vi "Calculate Counter And Protections Main Incoming.vi"(0 "Incoming Frames":T5[](array[typedef]) {"Protection Configurations"."CRC Channels"."Data Type" items=["Signed", "Unsigned", "IEEE Float"]}, 1 "TimeStamp.Ref":T1, 2 "TimeDiff.Ref":T1, 5 "Incoming Values in":T4, 7 "data":T2[](array[typedef]) {"payload" format="%x"; "timestamp" format="%<%.7X\n%x>T"; "type" items=["CAN Data"=0, "CAN Remote"=1, "CAN Bus Error"=2, "CAN 2.0 Data"=8, "CAN FD Data"=16, "CAN FD+BRS Data"=24, "J1939 Data"=192, "Delay"=224, "Log Trigger"=225, "Start Trigger"=226]; "identifier" format="%x"}, 11 "error in (no error)":errorcluster, 12 "IncomingSignals.Ref":T1, 13 "CtrandProtctnVld.Ref":T1, 14 "IncomingProtCtr.Ref":T1) -> (6 "Incoming Values out":T4, 15 "error out":errorcluster)   [LabVIEW 2024, in "Protection and Counter Support Engine.lvlib"]
uses:
  Protection and Counter Support Engine.lvlib
  Types/RT Frame Incoming Values.ctl
  Types/RT Frame Settings.ctl
  Shared/Types/Exported Frame Type.ctl
  Types/RT Protection Configuration.ctl
  Shared/Types/Protection Type.ctl
  Shared/Types/XNET Signal Configuration.ctl
  Shared/Types/Exported Counter Settings.ctl
  Shared/Types/Exported Event Trigger Type.ctl
  <vilib>/xnet/xnet.llb/XNET Frame CAN.ctl
  <vilib>/xnet/xnet.llb/XNET Frame Type CAN.ctl
  <vilib>/NI/NIVS Inline Async API/_Data Access Engine/Data Access Engine/Types/Write.DVR.ctl
  <vilib>/NI/NIVS Inline Async API/_Data Access Engine/Access Type Classes/Write/Write.lvclass
  <vilib>/NI/NIVS Inline Async API/_Data Access Engine/Access Type Classes/Write/Write.lvclass/Write.ctl
  <vilib>/NI/NIVS Inline Async API/_Data Access Engine/Data Access Engine/Methods/Write.Data.vi
  Calculate Protection Value.vi
  <vilib>/NI/NIVS Inline Async API/_Data Access Engine/Access Type Classes/Write/Write.ProcessData.vi
  Get Protection Signals.vi
  <vilib>/NI/NIVS Inline Async API/_Data Access Engine/Access Type Classes/Write/Write.Buffer.vi
  <vilib>/NI/NIVS Inline Async API/_Data Access Engine/Access Type Classes/Write/Write.Commit.vi
  <vilib>/xnet/xnet.llb/XNET Convert (Frame CAN to Signal).vi
  <vilib>/xnet/xnet.llb/XNET Convert (Signal to Frame Raw).vi
  <vilib>/NI/NIVS Inline Async API/_Data Access Engine/Data Access Engine/Data Access Engine.lvclass
  Shared/Protection and Counter Support Shared.lvlib
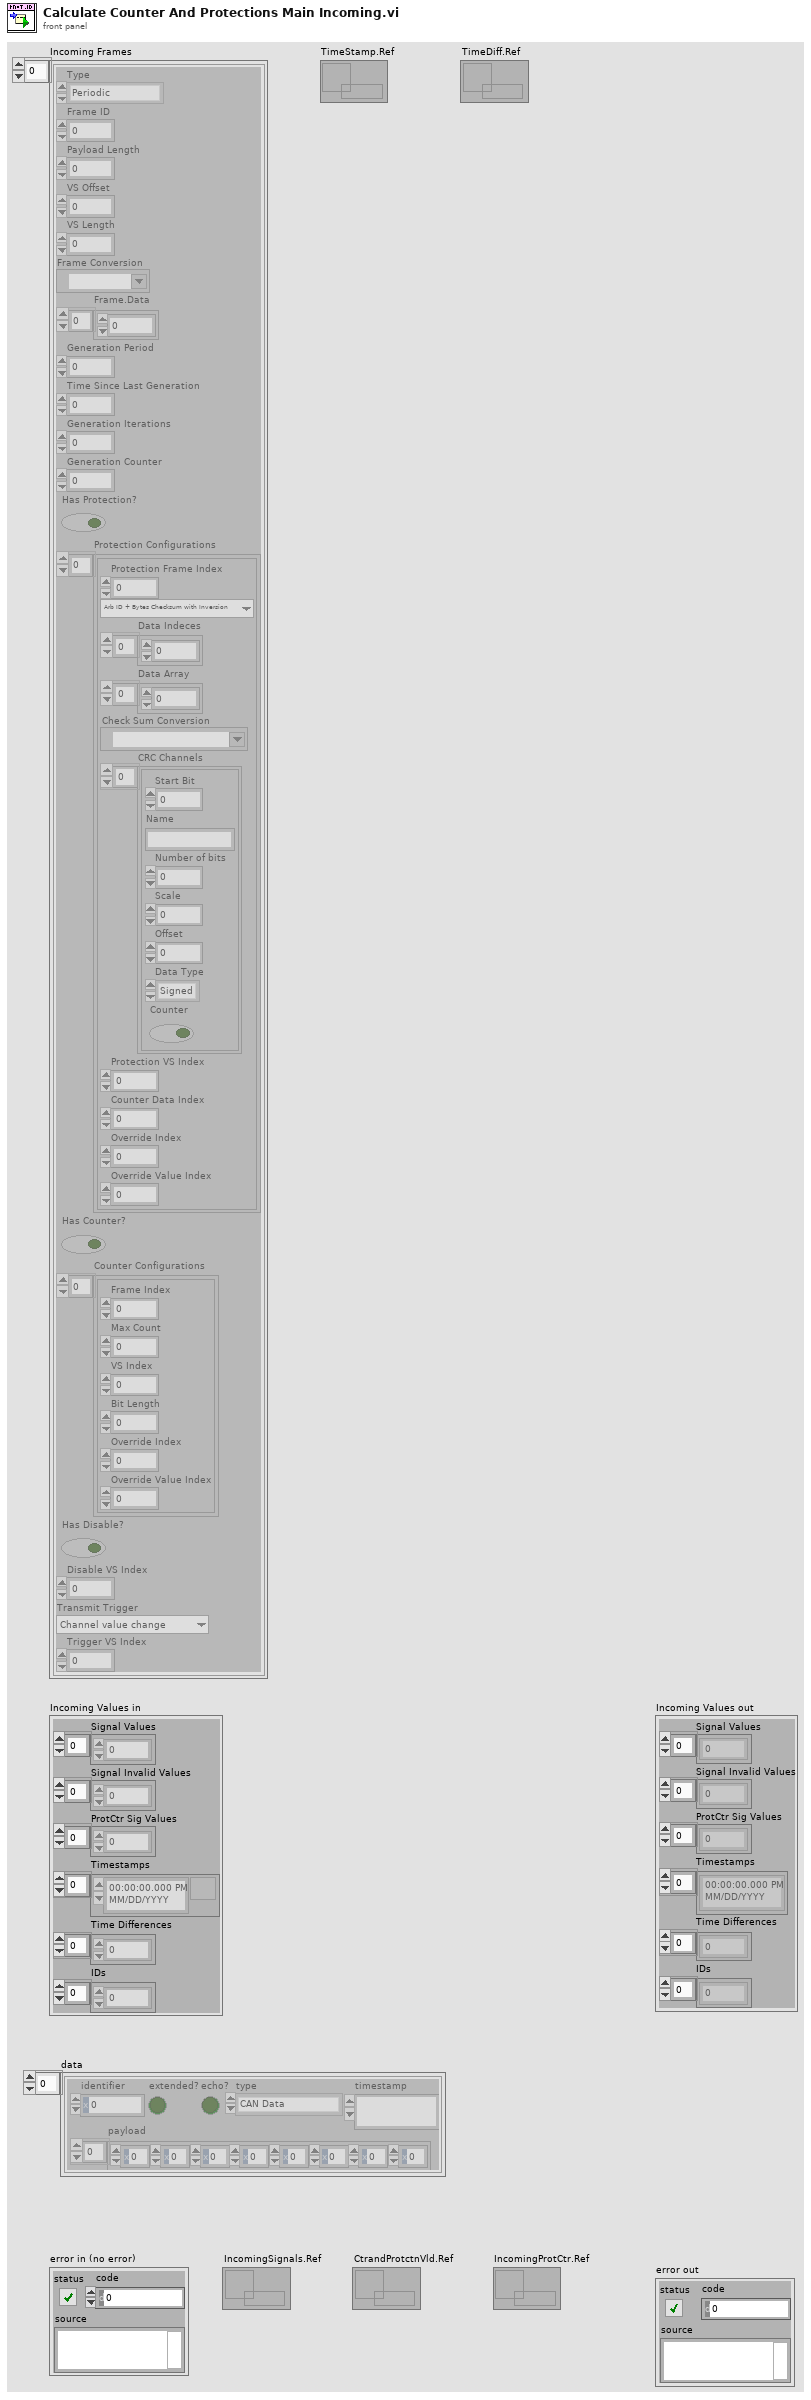
[diagram p1: front panel]
types:
  T1 = typedef "Data Access Engine.lvlib/Data Access Engine.lvclass/Write.DVR.ctl" = refnum<data-value>
  T2 = typedef "XNET Frame CAN.ctl" = cluster{"timestamp":timestamp, "payload":u8[], "identifier":u32, "type":T3, "extended?":bool, "echo?":bool}
  T3 = typedef "XNET Frame Type CAN.ctl" = u8
  T4 = typedef "Protection and Counter Support Engine.lvlib/RT Frame Incoming Values.ctl" = cluster{"Signal Values":dbl[], "Signal Invalid Values":dbl[], "ProtCtr Sig Values":dbl[], "Timestamps":timestamp[], "Time Differences":dbl[], "IDs":u32[]}
  T5 = typedef "Protection and Counter Support Engine.lvlib/RT Frame Settings.ctl" = cluster{"Type":T6, "Frame ID":u32, "Payload Length":u32, "VS Offset":i32, "VS Length":i32, "Frame Conversion":refnum<k21>, "Frame.Data":dbl[], "Generation Period":u32, "Time Since Last Generation":u32, "Generation Iterations":u32, "Generation Counter":u32, "Has Protection?":bool, "Protection Configurations":T7[], "Has Counter?":bool, "Counter Configurations":T10[], "Has Disable?":bool, "Disable VS Index":i32, "Transmit Trigger":T11, "Trigger VS Index":i32}
  T6 = typedef "Protection and Counter Support Shared.lvlib/Exported Frame Type.ctl" = enum16{"Periodic", "Event", "Periodic/Event"}
  T7 = typedef "Protection and Counter Support Engine.lvlib/RT Protection Configuration.ctl" = cluster{"Protection Frame Index":i32, "Protection Type":T8, "Data Indeces":i32[], "Data Array":dbl[], "Check Sum Conversion":refnum<k21>, "CRC Channels":T9[], "Protection VS Index":i32, "Counter Data Index":i32, "Override Index":i32, "Override Value Index":i32}
  T8 = typedef "Protection and Counter Support Shared.lvlib/Protection Type.ctl" = enum16{"Arb ID + Bytes Checksum with Inversion", "Arb ID + Bytes CRC with Inversion", "Reversed Raw Signal Checksum with Inversion", "Concatenated Two's Compliment"}
  T9 = typedef "Protection and Counter Support Shared.lvlib/XNET Signal Configuration.ctl" = cluster{"Start Bit":i32, "Name":string, "Number of bits":i32, "Scale":dbl, "Offset":dbl, "Data Type":u32, "Counter":bool}
  T10 = typedef "Protection and Counter Support Shared.lvlib/Exported Counter Settings.ctl" = cluster{"Frame Index":i32, "Max Count":dbl, "VS Index":i32, "Bit Length":i64, "Override Index":i32, "Override Value Index":i32}
  T11 = typedef "Protection and Counter Support Shared.lvlib/Exported Event Trigger Type.ctl" = enum16{"Channel value change", "Trigger channel (not zero)", "Channel value change or trigger channel (not zero)", "Trigger channel (any value change)", "Channel value change or trigger channel (any value change)"}
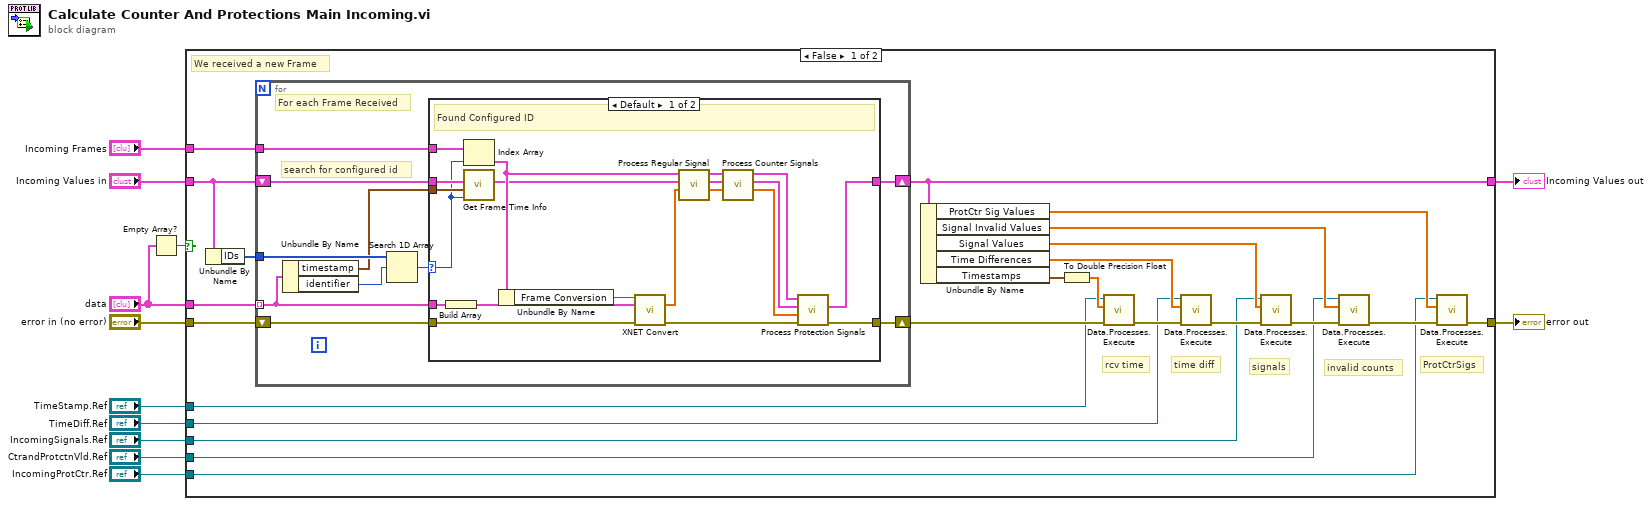
[diagram p0: block diagram]
diagram:
  n1 = Empty Array?(array="data") -> (empty?=w2:bool)
  n2 = case shown="False" w2 {
    tunnel: "data" -> [w33 _]
    tunnel: "error in (no error)" -> [w35 w69]
    tunnel: [w27 w69] -> w1
    tunnel: "TimeStamp.Ref" -> [w20 _]
    tunnel: "TimeDiff.Ref" -> [w19 _]
    tunnel: "IncomingSignals.Ref" -> [w18 _]
    tunnel: "CtrandProtctnVld.Ref" -> [w17 _]
    tunnel: "IncomingProtCtr.Ref" -> [w16 _]
    tunnel: "Incoming Frames" -> [w15 _]
    tunnel: "Incoming Values in" -> [w14 w68]
    tunnel: [w13 w68] -> w10
    frame False {
      # "ProtCtrSigs"
      # "time diff"
      # "signals"
      # "invalid counts"
      # "rcv time"
      # "We received a new Frame"
      n3 = Unbundle By Name(w14) -> ("IDs"=w21:u32[])
      n4 = for {
        tunnel: w33 -> [w38] mode=indexing
        shift-right: [w44] -> w32
        shift-left: w35 -> [w45]
        tunnel: w21 -> [w43]
        shift-right: [w39] -> w13
        shift-left: w14 -> [w40]
        tunnel: w15 -> [w37]
        # "search for configured id"
        # "For each Frame Received"
        n5 = Unbundle By Name(w38) -> ("timestamp"=w36:timestamp, "identifier"=w42:u32)
        n6 = Search 1D Array(1D array=w43, element=w42) -> (index of element=w41:i32)  [unwired: 1 in]
        n7 = case shown="Default" w41 {
          selector: w41 -> [w46 _]
          tunnel: w45 -> [w61 w67]
          tunnel: [w65 w67] -> w44
          tunnel: w37 -> [w63 _]
          tunnel: w36 -> [w47 _]
          tunnel: w40 -> [w52 w66]
          tunnel: [w56 w66] -> w39
          tunnel: w38 -> [w54 _]
          frame Default {
            # "Found Configured ID"
            n8 = Build Array(w54) -> (w53:T2[])
            n9 = Index Array(array=w63, index=w46) -> (element=w55:T5)
            n10 = call "Get Frame Time Info.vi"("Frame Index"=w46, "Current Time Stamp"=w47, "Settings.Incoming Values"=w52) -> ("Settings.Incoming Values out"=w51:T4)  [unwired: 8 in]
            n11 = Unbundle By Name(w55) -> ("Frame Conversion"=w62:refnum<k21>)
            n12 = call-poly <vilib>:"XNET Convert.vi"("session in"=w62, "frame data"=w53, "error in (no error)"=w61) -> ("signal data"=w49:dbl[], "error out"=w60:errorcluster)  [unwired: 10 in, 1 out]
            n13 = call "Process Regular Signal.vi"("Values Received"=w49, "Incoming Values In"=w51, "Frame Settings In"=w55) -> ("Values Received out"=w50:dbl[], "Incoming Values Out"=w57:T4, "Frame Settings Out"=w59:T5)  [unwired: 6 in]
            n14 = call "Process Counter Signals.vi"("Values Received"=w50, "Incoming Values In"=w57, "Frame Settings In"=w59) -> ("Values Received out"=w48:dbl[], "Incoming Values Out"=w64:T4, "Frame Settings Out"=w58:T5)  [unwired: 6 in]
            n15 = call "Process Protection Signals.vi"("Frame Settings In"=w58, "Incoming Values In"=w64, "Values Received"=w48, "error in (no error)"=w60) -> ("Incoming Values Out"=w56:T4, "error out"=w65:errorcluster)  [unwired: 4 in, 1 out]
          }
          frame -1 {
            # "Configured ID not Found"
          }
        }
      }
      n16 = Unbundle By Name(w13) -> ("ProtCtr Sig Values"=w24:dbl[], "Signal Invalid Values"=w25:dbl[], "Signal Values"=w26:dbl[], "Time Differences"=w22:dbl[], "Timestamps"=w23:timestamp[])
      n17 = To Double Precision Float(number=w23) -> (double precision float=w34:dbl[])
      n18 = call-poly <vilib>:"Data.Processes.Execute.vi"("error in (no error)"=w32, "Values"=w34, "Ref"=w20) -> ("error out"=w31:errorcluster)  [unwired: 8 in]
      n19 = call-poly <vilib>:"Data.Processes.Execute.vi"("error in (no error)"=w31, "Values"=w22, "Ref"=w19) -> ("error out"=w30:errorcluster)  [unwired: 8 in]
      n20 = call-poly <vilib>:"Data.Processes.Execute.vi"("error in (no error)"=w30, "Values"=w26, "Ref"=w18) -> ("error out"=w29:errorcluster)  [unwired: 8 in]
      n21 = call-poly <vilib>:"Data.Processes.Execute.vi"("error in (no error)"=w29, "Values"=w25, "Ref"=w17) -> ("error out"=w28:errorcluster)  [unwired: 8 in]
      n22 = call-poly <vilib>:"Data.Processes.Execute.vi"("error in (no error)"=w28, "Values"=w24, "Ref"=w16) -> ("error out"=w27:errorcluster)  [unwired: 8 in]
    }
    frame True {
      # "No Frame Received"
    }
  }
  "Incoming Values out" <- w10
  "error out" <- w1
